vi "RSNRPZ Set Burst Chopper State.vi"(8 "error in (no error)":errorcluster, 9 "BurstAv Chopper (T: On)":bool=TRUE, 10 "Channel (1)":i32=1, 11 "VISA session":refnum<visa-resource-name> caption="VISA resource name") -> (0 "error out":errorcluster, 3 "dup VISA session":refnum<visa-resource-name> caption="VISA resource name")   [LabVIEW 2010]
doc: "This VI enables or disables the chopper in BurstAv mode. Disabling the chopper is only good for fast but unexact and noisy measurements. If the chopper is disabled, averaging is ignored internally also disabled.\n\nRemote-control command(s):\nSENSe:POWer:BURSt:CHOPper:STATe"
uses:
  rsnrpz_32.dll
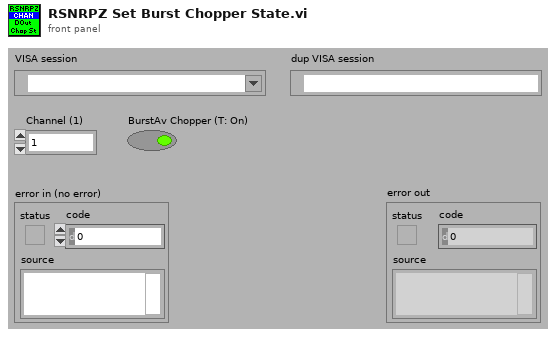
[diagram p1: front panel]
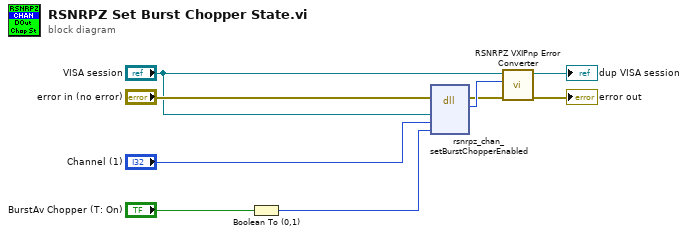
[diagram p0: block diagram]
diagram:
  n1 = Boolean To (0,1)(Boolean="BurstAv Chopper (T: On)") -> (0, 1=w6:i16)
  n2 = dll-call lib="rsnrpz_32.dll" fn="rsnrpz_chan_setBurstChopperEnabled"(error in="error in (no error)", "Instrument Handle"="VISA session", "Channel"="Channel (1)", "BurstAv Chopper"=w6) -> (error out=w5:errorcluster, "Status"=w8:i32)  [unwired: 5 in, 1 out]
  n3 = call <instrlib>:"RSNRPZ VXIPnp Error Converter.vi"("error in"=w5, "VXIPnp error code"=w8, "VISA session"="VISA session") -> ("error out"=→"error out":errorcluster, "dup VISA session"=→"dup VISA session":refnum<visa-resource-name>)  [unwired: 7 in]
